vi "Exit Multi Frame Structure.vi"(0 "Diagram in":refnum<vi>, 5 "Outputs":refnum<vi>[][](array[refnum]), 11 "error in (no error)":errorcluster) -> (4 "Diagram out":refnum<vi>, 6 "Outputs":refnum<vi>[](array[refnum]), 15 "error out":errorcluster)   [LabVIEW 2015, in "Scripting.lvlib"]
doc: "Exits the Multi Frame Structure that owns <B>Diagram in</B>, supplying the structure's owning diagram at <B>Diagram out</B>."
uses:
  Scripting.lvlib
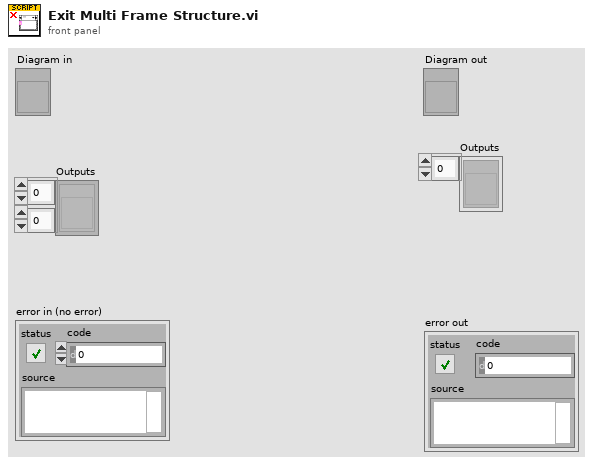
[diagram p1: front panel]
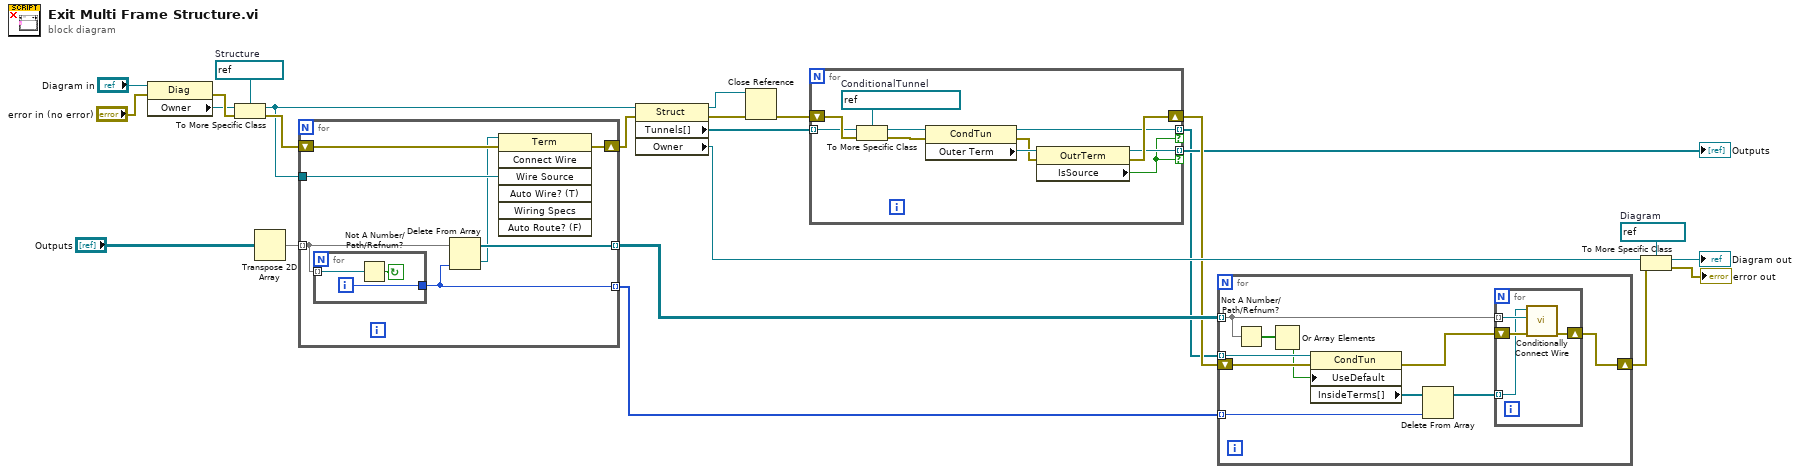
[diagram p0: block diagram]
diagram:
  w20 = refnum<vi> refnum  # Diagram
  w22 = refnum<vi> refnum  # Structure
  n1 = property class="Diag"(reference="Diagram in", error in="error in (no error)") -> (error out=w23:errorcluster, "Owner"=w21:refnum<vi>)  [unwired: 1 out]
  n2 = To More Specific Class(target class=w22, reference=w21, error in=w23) -> (specific class reference=w18:refnum<vi>, error out=w24:errorcluster)
  n3 = Transpose 2D Array(2D array="Outputs") -> (transposed array=w8:refnum<vi>[][])
  n4 = for {
    tunnel: w18 -> [w30]
    shift-right: [w29] -> w17
    shift-left: w24 -> [w31]
    tunnel: w8 -> [w25] mode=indexing
    tunnel: [w28] -> w16 mode=indexing
    tunnel: [w26] -> w3 mode=indexing
    n5 = for {
      tunnel: w25 -> [w32] mode=indexing
      tunnel: [w33] -> w26
      i -> [w33]
      stop <- w34 continue-if-true
      n6 = Not A Number/Path/Refnum?(number/path/refnum=w32) -> (NaN/Path/Refnum?=w34:bool)
    }
    n7 = Delete From Array(array=w25, index=w26) -> (deleted portion=w27:refnum<vi>, array with subset deleted=w28:refnum<vi>[])  [unwired: 1 in]
    n8 = invoke class="Term" method="Connect Wire"(reference=w27, error in=w31, "Wire Source"=w30) -> (error out=w29:errorcluster)  [unwired: 4 in, 6 out]
  }
  n9 = property class="Struct"(reference=w18, error in=w17) -> (reference out=w1:refnum<vi>, error out=w6:errorcluster, "Tunnels[]"=w7:refnum<vi>[], "Owner"=w19:refnum<vi>)
  n10 = Close Reference(reference=w1, error in (no error)=w6) -> (error out=w2:errorcluster)
  n11 = for {
    tunnel: w7 -> [w38] mode=indexing
    tunnel: [w41] -> w10 mode=indexing if=w35
    shift-right: [w42] -> w11
    shift-left: w2 -> [w45]
    tunnel: [w40] -> w9 mode=indexing if=w35
    w36 = refnum<vi> refnum  # ConditionalTunnel
    n12 = To More Specific Class(target class=w36, reference=w38, error in=w45) -> (specific class reference=w37:refnum<vi>, error out=w39:errorcluster)
    n13 = property class="CondTun"(reference=w37, error in=w39) -> (reference out=w40:refnum<vi>, error out=w43:errorcluster, "Outer Term"=w44:refnum<vi>)
    n14 = property class="OutrTerm"(reference=w44, error in=w43) -> (reference out=w41:refnum<vi>, error out=w42:errorcluster, "IsSource"=w35:bool)
  }
  "Outputs" <- w10
  n15 = for {
    tunnel: w9 -> [w54] mode=indexing
    shift-right: [w55] -> w12
    shift-left: w11 -> [w53]
    tunnel: w16 -> [w49] mode=indexing
    tunnel: w3 -> [w46] mode=indexing
    n16 = Not A Number/Path/Refnum?(number/path/refnum=w49) -> (NaN/Path/Refnum?=w48:bool[])
    n17 = Or Array Elements(Boolean array=w48) -> (logical OR=w47:bool)
    n18 = property class="CondTun"(reference=w54, error in=w53, "UseDefault"=w47) -> (error out=w52:errorcluster, "InsideTerms[]"=w51:refnum<vi>[])  [unwired: 1 out]
    n19 = Delete From Array(array=w51, index=w46) -> (array with subset deleted=w50:refnum<vi>[])  [unwired: 1 in, 1 out]
    n20 = for {
      shift-right: [w58] -> w55
      shift-left: w52 -> [w59]
      tunnel: w50 -> [w56] mode=indexing
      tunnel: w49 -> [w57] mode=indexing
      n21 = call "Conditionally Connect Wire.vi"("error in (no error)"=w59, "Wire Source"=w57, "Terminal in"=w56) -> ("error out"=w58:errorcluster)  [unwired: 7 in, 1 out]
    }
  }
  n22 = To More Specific Class(target class=w20, reference=w19, error in=w12) -> (specific class reference=→"Diagram out":refnum<vi>, error out=→"error out":errorcluster)
